vi "p_meas_init.vi"(8 "error in (no error)":errorcluster, 10 "Numeric":i16, 11 "communication":i16(ring)=2 items=["USB - Nova2", "USB - Vega", "USB - USBI", "RS232", "GPIB"]) -> (0 "error out":errorcluster, 2 "OK ?":bool, 3 "dup Visa Session":refnum<visa-resource-name>)   [LabVIEW 2012]
doc: "PowerDemo.vi\nThe Demo enables power measurement and display results.\nVersion 1.00\nLast Updated 16 Mars 2005\n\nDemo Program Steps:\n \n1) The vi executes InitCom.vi to open the communication session.\nThe default is RS232,Port2,9600 bps and Address 10 for USB.\n\nYou have to select USB or RS232 Protocol and\nupdate these values for any change.\n\n2) The vi executes ConfMeasure.vi to Send \"FP\" (Force Power) to Device and \"SI\" (Send unIts) to receive the units\n\n3) The vi executes a loop of SendPower.vi to get measurements.\nWhen no Overrange value the vi add value to array for update\nstatistics values.\n\nIn case of Error:\nError Out contains the Error Number and the vi's name where the error occured.\n\nVISA Error Codes -10738077360 to -1073807231\nOphir Error Codes -1300 to 1340"
panel:
  out "Device Response 2":string="\r\n"
  out "Device Response":string="\r\n"
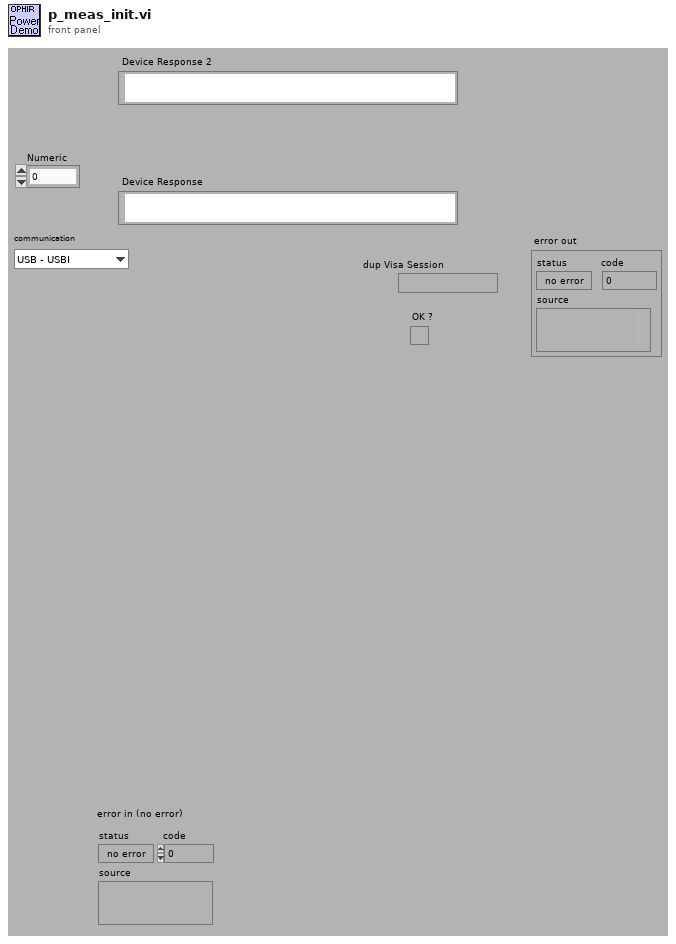
[diagram p1: front panel]
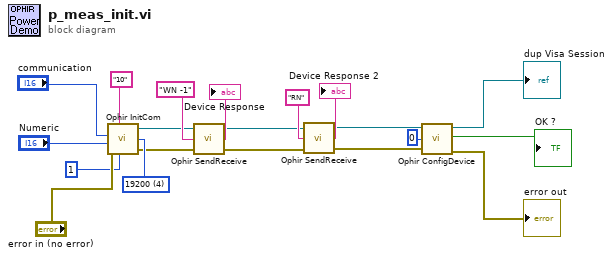
[diagram p0: block diagram]
diagram:
  w13 = i16 4 items=["300", "1200", "4800", "9600", "19200", "38400"] ("Baud Rate (3:9600)")
  n1 = call "Ophir InitCom.vi"("GPIB Address (10)"="10", "communication"="communication", "Numeric"="Numeric", "Port Number (default 2)"=i16 1, "error in (no error)"="error in (no error)", "Baud Rate (3:9600)"=w13) -> ("dup Visa Session"=w7:refnum<visa-resource-name>, "error out"=w8:errorcluster)  [unwired: 1 out]
  n2 = call "Ophir SendReceive.vi"("error in (no error)"=w8, "Command"="WN -1", "Visa Session"=w7) -> ("error out"=w2:errorcluster, "Frame Output"=→"Device Response":string, "dup Visa Session"=w4:refnum<visa-resource-name>)
  n3 = call "Ophir SendReceive.vi"("error in (no error)"=w2, "Command"="RN", "Visa Session"=w4) -> ("error out"=w1:errorcluster, "Frame Output"=→"Device Response 2":string, "dup Visa Session"=w3:refnum<visa-resource-name>)
  n4 = call "Ophir ConfigDevice.vi"("Visa Session"=w3, "Measure Choice (0:Power)"=u16 0, "error in (no error)"=w1) -> ("dup Visa Session"=→"dup Visa Session":refnum<visa-resource-name>, "OK ?"=→"OK ?":bool, "error out"=→"error out":errorcluster)  [unwired: 1 out]
